vi "Lookup Related Entities.vi"(6 "Relation":T1, 8 "error in (no error)":errorcluster, 9 "Primary ID":T3, 10 "Types":refnum<class "Type.lvclass">[](array[class]), 11 "Database in":refnum<class "Dummy DB.lvclass">) -> (0 "error out":errorcluster, 2 "Results":refnum<class "Result Row.lvclass">[](array[class]), 3 "Database out":refnum<class "Dummy DB.lvclass">)   [LabVIEW 2020, in "Scratchpad.lvlib" / "Dummy DB.lvclass"]
uses:
  Dummy DB.lvclass
  Conditum/Columns/Type/Type.lvclass
  Conditum/Entity ID.ctl
  Conditum/Columns/Relation/Relation Info.ctl
  Conditum/Relation Mapping.ctl
  Conditum/Result Row/Result Row.lvclass
  Conditum/Conditum.lvlib
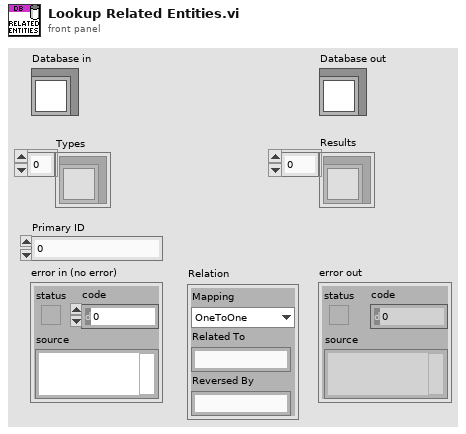
[diagram p1: front panel]
types:
  T1 = typedef "Conditum.lvlib/Relation Info.ctl" = cluster{"Mapping":T2, "Related To":string, "Reversed By":string}
  T2 = typedef "Conditum.lvlib/Relation Mapping.ctl" = enum16{"OneToOne", "OneToMany", "ManyToOne", "ManyToMany"}
  T3 = typedef "Conditum.lvlib/Entity ID.ctl" = i64
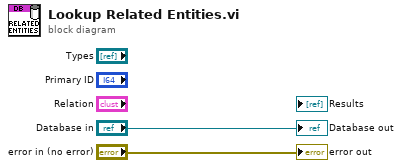
[diagram p0: block diagram]
diagram:
  "error out" <- "error in (no error)"
  "Database out" <- "Database in"
